vi "FPGA_SystemStart Async Agent.vi"(8 "error in":errorcluster) -> (0 "error out":errorcluster)   [LabVIEW 2017]
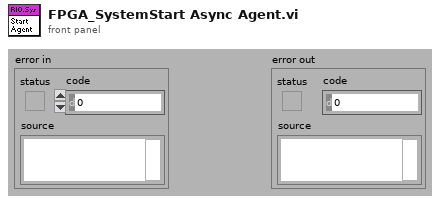
[diagram p1: front panel]
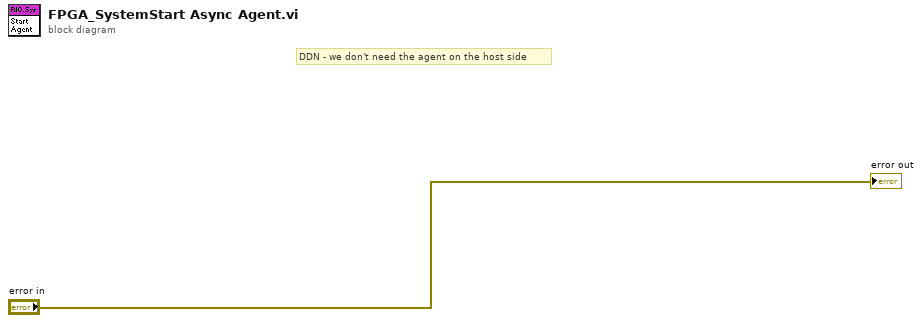
[diagram p0: block diagram]
diagram:
  # "DDN - we don't need the agent on the host side"
  "error out" <- "error in"
